vi "Define Columns.vi"(10 "Enum Array":refnum<vi>[](array[refnum])) -> (2 "Column Definition":T1[](array[typedef]) {"MinWidth" min=2 step=1; "AutoSizeMode" items=["None"=1, "ColumnHeader"=2, "AllCellsExceptHeader"=4, "AllCells"=6, "DisplayedCellsExceptHeader"=8, "DisplayedCells"=10, "Fill"=16]; "FillWeight" min=1 max=100})   [LabVIEW 2014, in "OPC UA Client editor node.lvclass"]
doc: "This VI defines the columns that will be used in the table. You can specify the column type and the dimensions if the columns."
uses:
  OPC UA Client editor node.lvclass
  <vilib>/NI/DCAF/Tag Editor Core/Table API/Column/Column Descriptor.ctl
  <vilib>/NI/DCAF/Tag Editor Core/Table API/Column/Column.lvclass
  <vilib>/NI/DCAF/Tag Editor Core/Table API/Column/Column Type.ctl
  <vilib>/NI/Tag Bus/tag/Data Type.ctl
  <vilib>/NI/DCAF/Tag Editor Core/Table API/Table Manager/Call Back Ref Type Def.ctl
  <vilib>/NI/DCAF/Tag Editor Core/Configuration Editor/Classes/Engine Parent/Engine Parent Editor Node.lvclass
  <vilib>/NI/DCAF/Tag Editor Core/Configuration Editor/Classes/Module editor node/module editor node.lvclass
  Callback Change Channel Name.vi
  Callback Change Direction.vi
  Callback Change Tag.vi
  Callback Change Node Path.vi
  Callback Change UA Data Type.vi
  <vilib>/NI/DCAF/Tag Editor Core/Table API/Mapping Column/Mapping Column.lvclass
  <vilib>/NI/DCAF/Tag Editor Core/Table API/String Column/String Column.lvclass
  <vilib>/NI/DCAF/Tag Editor Core/Table API/Listbox Enum Column/List Box Enum Column.lvclass
  <vilib>/NI/Tag Bus/tag/tag descriptor.lvclass
  <vilib>/NI/DCAF/Tag Editor Core/Table API/Table Manager/Table Manager.lvclass
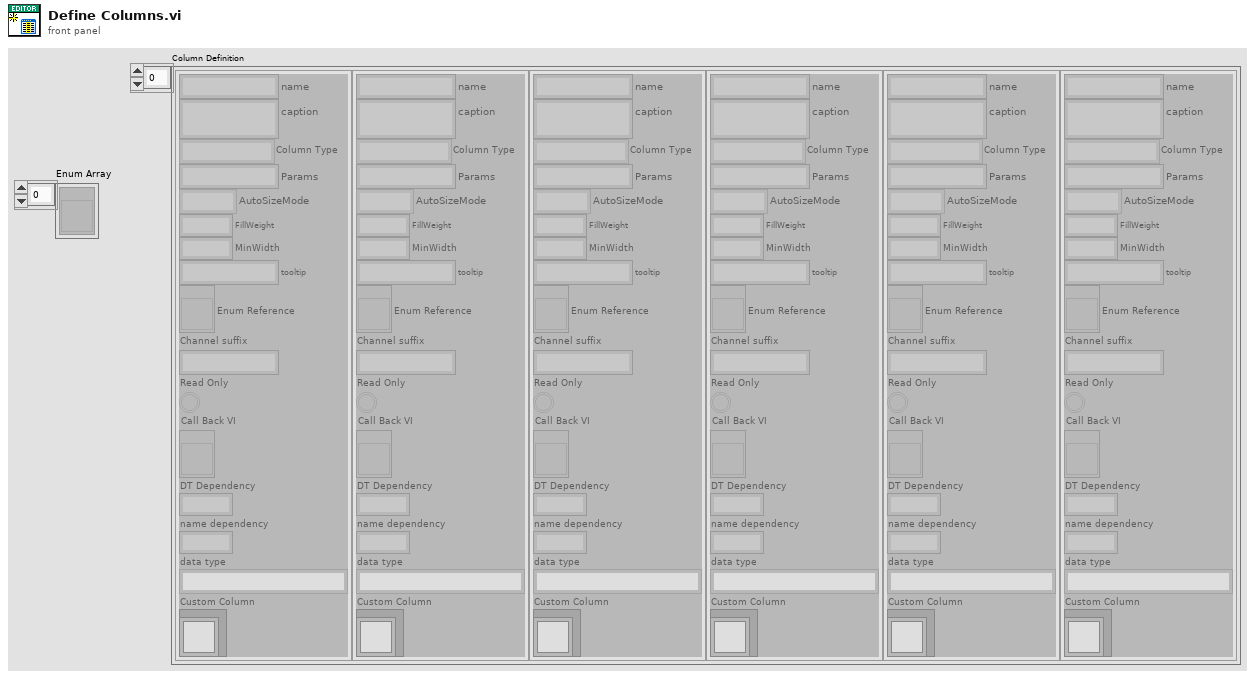
[diagram p1: front panel]
types:
  T1 = typedef "Table Manager.lvlib/Column.lvclass/Column Descriptor.ctl" = cluster{"name":string, "caption":string, "Column Type":T2, "Params":string, "AutoSizeMode":i32, "FillWeight":sgl, "MinWidth":u32, "tooltip":string, "Enum Reference":refnum<vi>, "Channel suffix":string, "Read Only":bool, "Call Back VI":T3, "DT Dependency":i32, "name dependency":i32, "data type":T4, "Custom Column":refnum<class "Column.lvclass">}
  T2 = typedef "Table Manager.lvlib/Column.lvclass/Column Type.ctl" = enum16{"String", "Mapping", "Enum", "Custom"}
  T3 = typedef "Table Manager.lvlib/Table Manager.lvclass/Call Back Ref Type Def.ctl" = refnum<vi>
  T4 = typedef "tag bus.lvlib/tag descriptor.lvclass/Data Type.ctl" = enum16{"Double", "Single", "I64", "I32", "I16", "I8", "U64", "U32", "U16", "U8", "Boolean", "String", "Array of Double", "Array of Single", "Array of I64", "Array of I32", "Array of I16", "Array of I8", "Array of U64", "Array of U32", "Array of U16", "Array of U8", "Array of Boolean", "Array of String"}
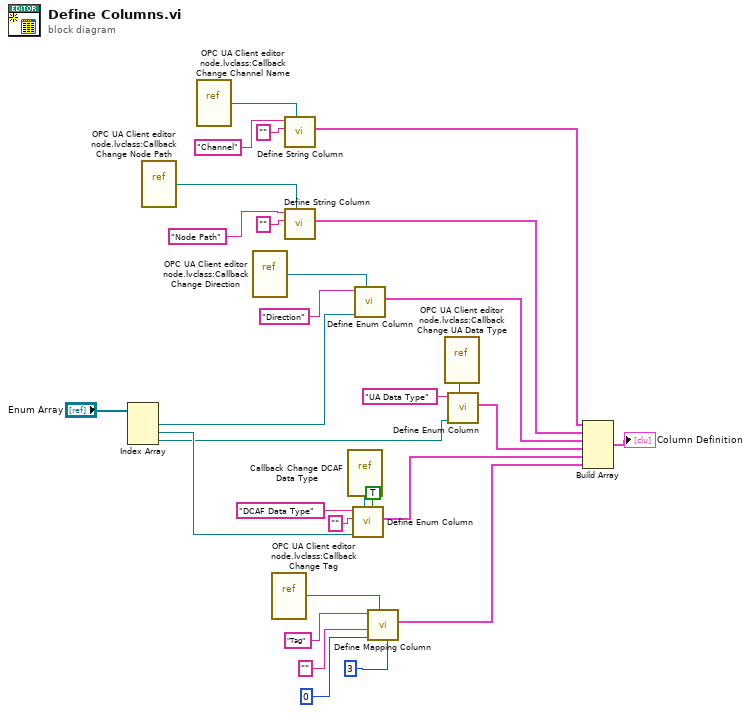
[diagram p0: block diagram]
diagram:
  n1 = Index Array(array="Enum Array") -> (element #1=w21:refnum<vi>, element #2=w18:refnum<vi>, element #3=w1:refnum<vi>)  [unwired: 3 in]
  n2 = vi-ref "OPC UA Client editor node.lvclass:Callback Change Node Path.vi"() -> (w10:refnum<vi>)
  n3 = vi-ref "OPC UA Client editor node.lvclass:Callback Change Channel Name.vi"() -> (w16:refnum<vi>)
  n4 = vi-ref "OPC UA Client editor node.lvclass:Callback Change Direction.vi"() -> (w15:refnum<vi>)
  n5 = vi-ref "OPC UA Client editor node.lvclass:Callback Change Tag.vi"() -> (w13:refnum<vi>)
  n6 = call <vilib>:"Define String Column.vi"("Call Back VI"=w16, "Caption"="", "Name"="Channel" ("name")) -> ("Column Descriptor out"=w9:T1)  [unwired: 8 in]
  n7 = call <vilib>:"Define String Column.vi"("Call Back VI"=w10, "Caption"="", "Name"="Node Path" ("name")) -> ("Column Descriptor out"=w8:T1)  [unwired: 8 in]
  n8 = vi-ref "Callback Change DCAF Data Type.vi"() -> (w14:refnum<vi>)
  n9 = call <vilib>:"Define Enum Column.vi"("Read Only (F)"=TRUE, "Call Back VI"=w14, "Enum Reference"=w18, "Caption"="", "Name"="DCAF Data Type" ("name")) -> ("Column Descriptor out"=w5:T1)  [unwired: 6 in]
  n10 = call <vilib>:"Define Enum Column.vi"("Call Back VI"=w15, "Enum Reference"=w21, "Name"="Direction" ("name")) -> ("Column Descriptor out"=w17:T1)  [unwired: 8 in]
  n11 = call <vilib>:"Define Mapping Column.vi"("DT Dependency (-1)"=3 ("DT Dependency"), "Call Back VI"=w13, "name dependency"=0, "Channel suffix"="" ("string"), "name"="Tag") -> ("Column Descriptor out"=w6:T1)  [unwired: 6 in]
  n12 = vi-ref "OPC UA Client editor node.lvclass:Callback Change UA Data Type.vi"() -> (w3:refnum<vi>)
  n13 = call <vilib>:"Define Enum Column.vi"("Call Back VI"=w3, "Enum Reference"=w1, "Name"="UA Data Type" ("name")) -> ("Column Descriptor out"=w2:T1)  [unwired: 8 in]
  n14 = Build Array(w9, w8, w17, w2, w5, w6) -> (→"Column Definition":T1[])
